vi "Oxford Get Data.vi"(2 "Point #":i32, 3 "Command String":string, 4 "Instrument Address":refnum<visa-resource-name>) -> (0 "Stop":bool, 1 "Output":dbl[](array[numeric]) format="%.2f")   [LabVIEW 2025]
doc: "This VI reads the sample output of the Lakeshore DRC 93C or 82C temperature controller. The output is an array consisting of the single reading. The input is the numeric GPIB address.\nScott Hannahs, F. Bitter National Magnet Lab, 1993\nAuthor: Scott Hannahs <sth@magnet.fsu.edu>\n\nThis software is licensed for use under the “MIT License\"\nCopyright (c) 2025 Scott Hannahs, sth@sth@magnet.sthnet.net\n\nPermission is hereby granted, free of charge, to any person obtaining a copy of this software and associated documentation files (the \"Software\"), to deal in the Software without restriction, including without limitation the rights to use, copy, modify, merge, publish, distribute, sublicense, and/or sell copies of the Software, and to permit persons to whom the Software is furnished to do so, subject to the following conditions: The above copyright notice and this permission notice shall be included in all copies or substantial portions of the Software.\n\nTHE SOFTWARE IS PROVIDED \"AS IS\", WITHOUT WARRANTY OF ANY KIND, EXPRESS OR IMPLIED, INCLUDING BUT NOT LIMITED TO THE WARRANTIES OF MERCHANTABILITY, FITNESS FOR A PARTICULAR PURPOSE AND NONINFRINGEMENT. IN NO EVENT SHALL THE AUTHORS OR COPYRIGHT HOLDERS BE LIABLE FOR ANY CLAIM, DAMAGES OR OTHER LIABILITY, WHETHER IN AN ACTION OF CONTRACT, TORT OR OTHERWISE, ARISING FROM, OUT OF OR IN CONNECTION WITH THE SOFTWARE OR THE USE OR OTHER DEALINGS IN THE SOFTWARE."
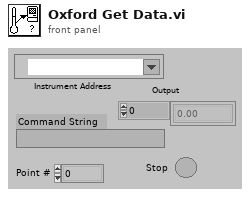
[diagram p1: front panel]
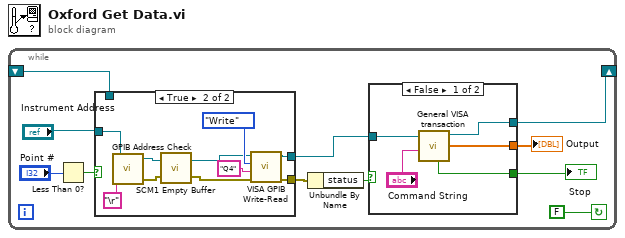
[diagram p0: block diagram]
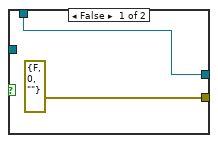
[diagram p2: hidden frame]
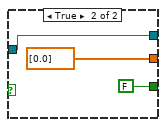
[diagram p3: hidden frame]
diagram:
  n1 = while {
    shift-left: _ -> [w8]
    shift-right: [w7] -> _
    stop <- FALSE continue-if-true
    n2 = Less Than 0?(x="Point #") -> (x < 0?=w9:bool)
    n3 = case shown="True" w9 {
      tunnel: "Instrument Address" -> [_ w20]
      tunnel: [errorcluster {"status"=FALSE, "code"=0, "source"=""} ("error out") w21] -> w4
      tunnel: [w12 w19] -> w6
      tunnel: w8 -> [w12 _]
      frame False {
      }
      frame True {
        n4 = call "GPIB Address Check.vi"("Instrument Address"=w20, "Term Char"="\r") -> ("dup VISA session"=w18:refnum<visa-resource-name>, "error out"=w17:errorcluster)  [unwired: 1 out]
        n5 = call "SCM1 Empty Buffer.vi"("error in (no error)"=w17, "VISA Resource Name"=w18) -> ("error out"=w15:errorcluster, "dup VISA Resource Name"=w16:refnum<visa-resource-name>)
        n6 = call "VISA GPIB Write-Read.vi"("error in (no error)"=w15, "Command"="Q4" ("String to Write"), "Action"=enum16{"Write", "Read", "Write & Read"}."Write", "VISA resource name"=w16) -> ("error out"=w21:errorcluster, "dup VISA Session"=w19:refnum<visa-resource-name>)  [unwired: 4 in, 2 out]
      }
    }
    n7 = Unbundle By Name(w4) -> ("status"=w11:bool)
    n8 = case shown="False" w11 {
      tunnel: w6 -> [w28 w30]
      tunnel: [w26 dbl[] [0.0]] -> w5
      tunnel: [w27 w30] -> w7
      tunnel: [w25 FALSE ("Stop")] -> w3
      frame False {
        n9 = call "General VISA transaction.vi"("Command String"="Command String", "VISA Session"=w28) -> ("Measurement"=w26:dbl[], "dup VISA Session"=w27:refnum<visa-resource-name>, "Stop"=w25:bool)  [unwired: 4 in, 3 out]
      }
      frame True {
      }
    }
    "Stop" <- w3
    "Output" <- w5
  }
